vi "Set Desaccade Manipulator.vi"(8 "error in (no error)":errorcluster, 10 "Desaccade Manipulator.lvclass":refnum<class "Desaccade Manipulator.lvclass">, 11 "Impulse Manager in":refnum<class "Impulse Manager.lvclass">) -> (0 "error out":errorcluster, 3 "Impulse Manager out":refnum<class "Impulse Manager.lvclass">)   [LabVIEW 2013, in "Impulse Manager.lvclass"]
uses:
  Impulse Manager.lvclass
  Desaccade Manipulator/Desaccade Manipulator.lvclass
  Impulse Manager.lvclass/Impulse Manager.ctl
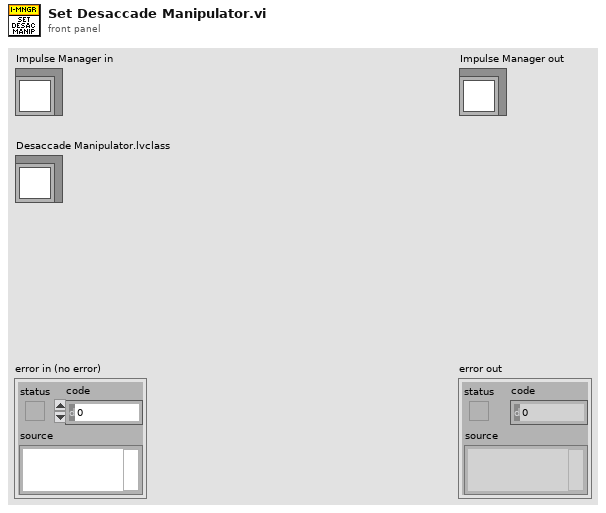
[diagram p1: front panel]
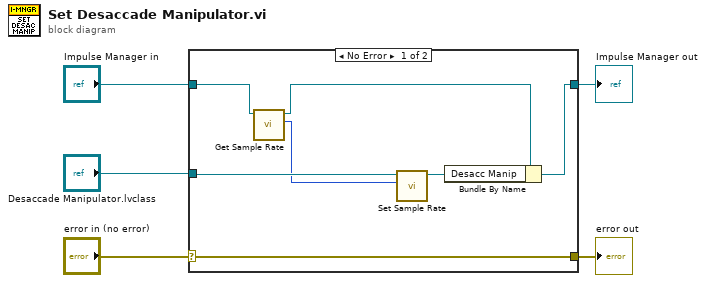
[diagram p0: block diagram]
diagram:
  n1 = case shown="No Error" "error in (no error)" {
    selector: "error in (no error)" -> [w12 w13]
    tunnel: [w12 w13] -> w4
    tunnel: [w11 w14] -> w2
    tunnel: "Impulse Manager in" -> [w8 w14]
    tunnel: "Desaccade Manipulator.lvclass" -> [w9 _]
    frame No Error {
      n2 = call-dynamic "Get Sample Rate.vi"("Impulse Manager in"=w8) -> ("Sample Rate"=w6:i32, "Impulse Manager out"=w7:refnum<class "Impulse Manager.lvclass">)  [unwired: 8 in, 1 out]
      n3 = call-dynamic "Set Sample Rate.vi"("Sample Rate"=w6, "Desaccade Manipulator in"=w9) -> ("Desaccade Manipulator out"=w10:refnum<class "Desaccade Manipulator.lvclass">)  [unwired: 8 in, 1 out]
      n4 = Bundle By Name(cluster=w7, "Desacc Manip"=w10) -> (w11:refnum<class "Impulse Manager.lvclass">)
    }
    frame Error {
    }
  }
  "error out" <- w4
  "Impulse Manager out" <- w2
